vi "InitArmKinematics.vi"   [LabVIEW 2020]
doc: "Initializes the arm kinematics objects."
uses:
  <vilib>/robotics/Kinematics/DH Kinematic Parameters.ctl
  <vilib>/robotics/Kinematics/Link/Joint Type.ctl
  <vilib>/robotics/Kinematics/DH Dynamic Parameters.ctl
  <vilib>/Analysis/Matrix/Datatypes/RealMatrix.ctl
  <vilib>/robotics/Kinematics/RotateX.vi
  <vilib>/robotics/Kinematics/RotateY.vi
  <vilib>/robotics/Kinematics/RotateZ.vi
  <vilib>/Analysis/baseanly.llb/A x B.vi
  <vilib>/Analysis/baseanly.llb/Real A x B.vi
  GlobalArm.vi
  <vilib>/robotics/Kinematics/Analytical/Initialize Generic Serial Arm.vi
  <vilib>/robotics/Kinematics/Robot/NI_Robotics_Serial Robot Arm.lvclass
  <vilib>/robotics/Kinematics/Link/NI_Robotics_Link.lvclass
  <vilib>/robotics/Kinematics/NI_Kinematics.lvlib
  <vilib>/robotics/Kinematics/Analytical/NI_Robotics_AnalyticKinematics.lvlib
  <vilib>/Analysis/Matrix/NI_Matrix.lvlib
types:
  T1 = typedef "DH Dynamic Parameters.ctl" = cluster{"mass":dbl, "gear ratio":dbl, "motor inertia":dbl, "center of gravity":dbl[], "viscous friction":dbl, "positive coulomb friction":dbl, "negative coulomb friction":dbl, "inertia matrix":T2}
  T2 = typedef "NI_Matrix.lvlib/RealMatrix.ctl" = dbl[][]
  T3 = typedef "DH Kinematic Parameters.ctl" = cluster{"twist angle":dbl, "length":dbl, "rotation angle":dbl, "offset distance":dbl, "joint type":T4, "joint coordinate offset":dbl}
  T4 = typedef "NI_Robotics_Link.lvclass/Joint Type.ctl" = enum16{"Revolute", "Prismatic"}
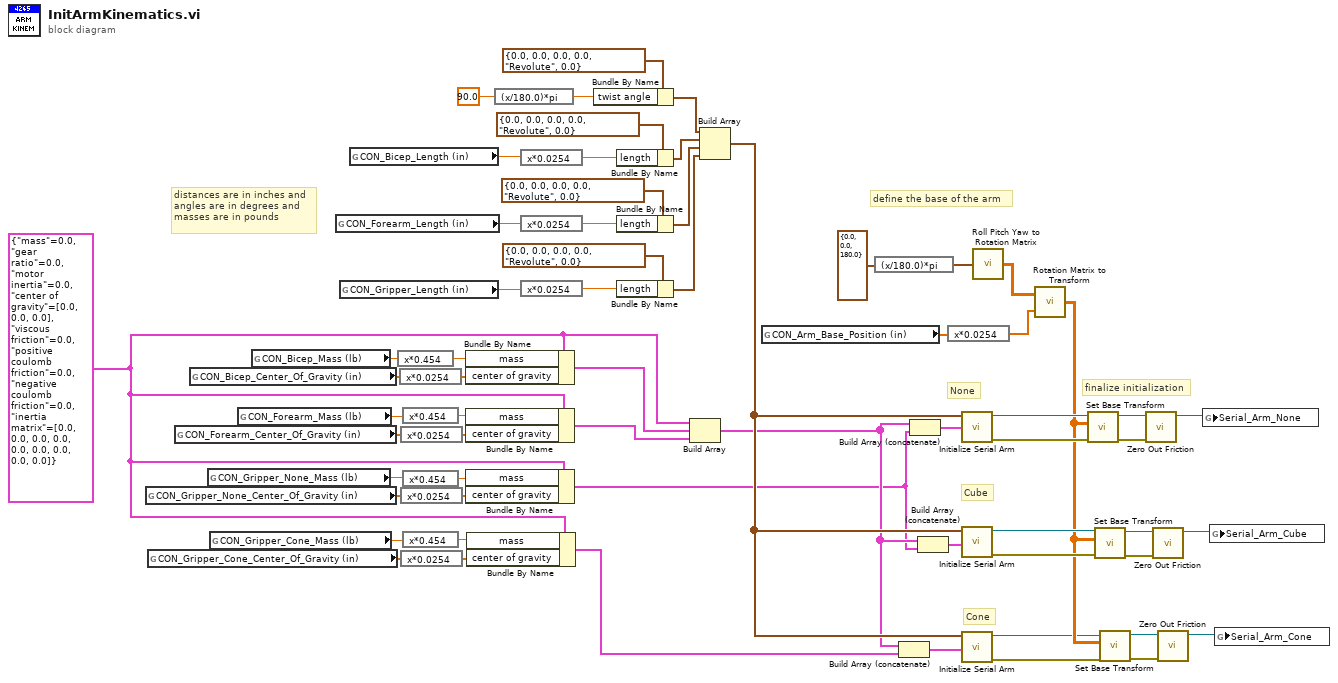
[diagram p0: block diagram]
diagram:
  w63 = T1 {"mass"=0.0, "gear ratio"=0.0, "motor inertia"=0.0, "center of gravity"=[0.0, 0.0, 0.0], "viscous friction"=0.0, "positive coulomb friction"=0.0, "negative coulomb friction"=0.0, "inertia matrix"=[[0.0, 0.0, 0.0], [0.0, 0.0, 0.0], [0.0, 0.0, 0.0]]} ("dynamic parameters")
  # "Cube"
  # "None"
  # "Cone"
  # "define the base of the arm"
  # "distances are in inches and\nangles are in degrees and\nmasses are in pounds"
  # "finalize initialization"
  n1 = global read "GlobalArm.vi" "CON_Gripper_None_Center_Of_Gravity (in)"() -> (w21:dbl[])
  n2 = global read "GlobalArm.vi" "CON_Gripper_Cone_Center_Of_Gravity (in)"() -> (w19:dbl[])
  n3 = global read "GlobalArm.vi" "CON_Forearm_Center_Of_Gravity (in)"() -> (w25:dbl[])
  n4 = global read "GlobalArm.vi" "CON_Bicep_Center_Of_Gravity (in)"() -> (w22:dbl[])
  n5 = global read "GlobalArm.vi" "CON_Gripper_None_Mass (lb)"() -> (w13:dbl)
  n6 = global read "GlobalArm.vi" "CON_Gripper_Cone_Mass (lb)"() -> (w11:dbl)
  n7 = global read "GlobalArm.vi" "CON_Forearm_Mass (lb)"() -> (w15:dbl)
  n8 = global read "GlobalArm.vi" "CON_Bicep_Mass (lb)"() -> (w17:dbl)
  n9 = global read "GlobalArm.vi" "CON_Forearm_Length (in)"() -> (w32:dbl)
  n10 = global read "GlobalArm.vi" "CON_Gripper_Length (in)"() -> (w34:dbl)
  n11 = global read "GlobalArm.vi" "CON_Bicep_Length (in)"() -> (w33:dbl)
  n12 = expression code="x*0.454" ("degrees to radians")(w17) -> (w16:dbl)
  n13 = expression code="x*0.0254" ("degrees to radians")(w22) -> (w23:dbl[])
  n14 = expression code="x*0.0254" ("degrees to radians")(w25) -> (w24:dbl[])
  n15 = expression code="x*0.0254" ("degrees to radians")(w21) -> (w20:dbl[])
  n16 = expression code="x*0.0254" ("degrees to radians")(w19) -> (w18:dbl[])
  n17 = expression code="x*0.454" ("degrees to radians")(w15) -> (w14:dbl)
  n18 = expression code="x*0.454" ("degrees to radians")(w13) -> (w12:dbl)
  n19 = expression code="x*0.454" ("degrees to radians")(w11) -> (w10:dbl)
  n20 = Bundle By Name(cluster=w63, "mass"=w16, "center of gravity"=w23) -> (w31:T1)
  n21 = Bundle By Name(cluster=w63, "mass"=w14, "center of gravity"=w24) -> (w30:T1)
  n22 = Bundle By Name(cluster=w63, "mass"=w12, "center of gravity"=w20) -> (w28:T1)
  n23 = Bundle By Name(cluster=w63, "mass"=w10, "center of gravity"=w18) -> (w27:T1)
  n24 = expression code="(x/180.0)*pi" ("degrees to radians")(90.0 ("twist angle")) -> (w51:dbl)
  n25 = expression code="x*0.0254" ("degrees to radians")(w33) -> (w56:dbl)
  n26 = expression code="x*0.0254" ("degrees to radians")(w32) -> (w38:dbl)
  n27 = expression code="x*0.0254" ("degrees to radians")(w34) -> (w37:dbl)
  n28 = Bundle By Name(cluster=T3 {"twist angle"=0.0, "length"=0.0, "rotation angle"=0.0, "offset distance"=0.0, "joint type"=enum."Revolute", "joint coordinate offset"=0.0} ("Link Parameters"), "twist angle"=w51) -> (w50:T3)
  n29 = Bundle By Name(cluster=T3 {"twist angle"=0.0, "length"=0.0, "rotation angle"=0.0, "offset distance"=0.0, "joint type"=enum."Revolute", "joint coordinate offset"=0.0} ("Link Parameters"), "length"=w56) -> (w55:T3)
  n30 = Bundle By Name(cluster=T3 {"twist angle"=0.0, "length"=0.0, "rotation angle"=0.0, "offset distance"=0.0, "joint type"=enum."Revolute", "joint coordinate offset"=0.0} ("Link Parameters"), "length"=w38) -> (w35:T3)
  n31 = Bundle By Name(cluster=T3 {"twist angle"=0.0, "length"=0.0, "rotation angle"=0.0, "offset distance"=0.0, "joint type"=enum."Revolute", "joint coordinate offset"=0.0} ("Link Parameters"), "length"=w37) -> (w36:T3)
  n32 = Build Array(w63, w31, w30) -> (w29:T1[])
  n33 = Build Array(w50, w55, w35, w36) -> (w45:T3[])
  n34 = global read "GlobalArm.vi" "CON_Arm_Base_Position (in)"() -> (w26:dbl[])
  n35 = expression code="(x/180.0)*pi" ("degrees to radians")(cluster{"roll":dbl, "pitch":dbl, "yaw":dbl} {"roll"=0.0, "pitch"=0.0, "yaw"=180.0} ("angles")) -> (w53:cluster{"roll":dbl, "pitch":dbl, "yaw":dbl})
  n36 = Build Array (concatenate)(w29, w27) -> (w46:T1[])
  n37 = Build Array (concatenate)(w29, w28) -> (w39:T1[])
  n38 = Build Array (concatenate)(w29, w28) -> (w47:T1[])
  n39 = expression code="x*0.0254" ("degrees to radians")(w26) -> (w52:dbl[])
  n40 = call-poly <vilib>:"Initialize Serial Arm.vi"("dynamic parameters"=w39, "kinematic parameters"=w45) -> ("error out"=w49:errorcluster, "serial arm out"=w48:refnum<class "NI_Robotics_Serial Robot Arm.lvclass">)  [unwired: 8 in]
  n41 = call-poly <vilib>:"Initialize Serial Arm.vi"("dynamic parameters"=w47, "kinematic parameters"=w45) -> ("error out"=w43:errorcluster, "serial arm out"=w44:refnum<class "NI_Robotics_Serial Robot Arm.lvclass">)  [unwired: 8 in]
  n42 = call-poly <vilib>:"Initialize Serial Arm.vi"("dynamic parameters"=w46, "kinematic parameters"=w45) -> ("error out"=w40:errorcluster, "serial arm out"=w41:refnum<class "NI_Robotics_Serial Robot Arm.lvclass">)  [unwired: 8 in]
  n43 = call <vilib>:"Roll Pitch Yaw to Rotation Matrix.vi"("angles"=w53) -> ("rotation matrix"=w54:T2)
  n44 = call <vilib>:"Rotation Matrix to Transform.vi"("translation vector"=w52, "rotation matrix"=w54) -> ("transform"=w42:T2)
  n45 = call <vilib>:"Set Base Transform.vi"("error in (no error)"=w49, "base transform"=w42, "serial arm in"=w48) -> ("error out"=w3:errorcluster, "serial arm out"=w4:refnum<class "NI_Robotics_Serial Robot Arm.lvclass">)  [unwired: 7 in]
  n46 = call <vilib>:"Set Base Transform.vi"("error in (no error)"=w43, "base transform"=w42, "serial arm in"=w44) -> ("error out"=w5:errorcluster, "serial arm out"=w6:refnum<class "NI_Robotics_Serial Robot Arm.lvclass">)  [unwired: 7 in]
  n47 = call <vilib>:"Set Base Transform.vi"("error in (no error)"=w40, "base transform"=w42, "serial arm in"=w41) -> ("error out"=w1:errorcluster, "serial arm out"=w2:refnum<class "NI_Robotics_Serial Robot Arm.lvclass">)  [unwired: 7 in]
  n48 = call <vilib>:"Zero Out Friction.vi"("error in (no error)"=w3, "serial arm in"=w4) -> ("serial arm out"=w9:refnum<class "NI_Robotics_Serial Robot Arm.lvclass">)  [unwired: 8 in, 1 out]
  n49 = call <vilib>:"Zero Out Friction.vi"("error in (no error)"=w5, "serial arm in"=w6) -> ("serial arm out"=w8:refnum<class "NI_Robotics_Serial Robot Arm.lvclass">)  [unwired: 8 in, 1 out]
  n50 = call <vilib>:"Zero Out Friction.vi"("error in (no error)"=w1, "serial arm in"=w2) -> ("serial arm out"=w7:refnum<class "NI_Robotics_Serial Robot Arm.lvclass">)  [unwired: 8 in, 1 out]
  n51 = global write "GlobalArm.vi" "Serial_Arm_None"(w9) -> ()
  n52 = global write "GlobalArm.vi" "Serial_Arm_Cube"(w8) -> ()
  n53 = global write "GlobalArm.vi" "Serial_Arm_Cone"(w7) -> ()
